vi "waypoint.vi"(11 "Vision Data":dbl[](array[numeric])) -> (3 "Waypoints":dbl[][](array[numeric]))   [LabVIEW 2018]
panel:
  in  "Multiplier":dbl format="%#_13g"
  out "XY Graph":cluster{dbl[], dbl[]}[](graph)
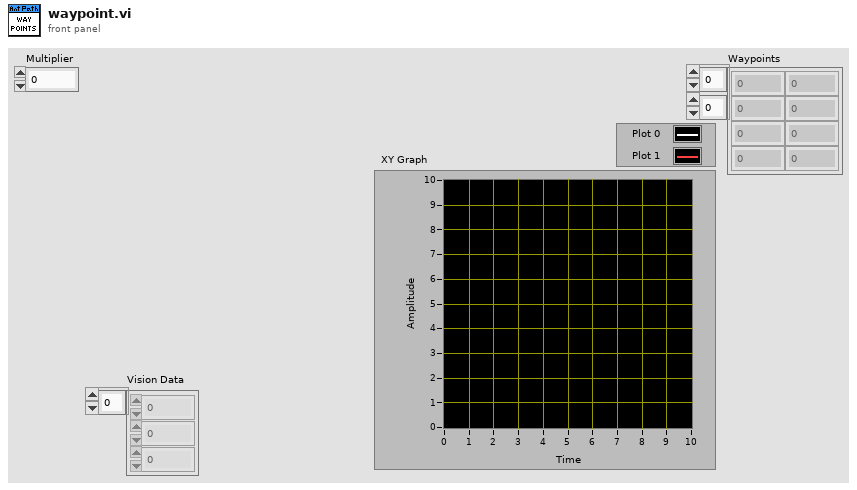
[diagram p1: front panel]
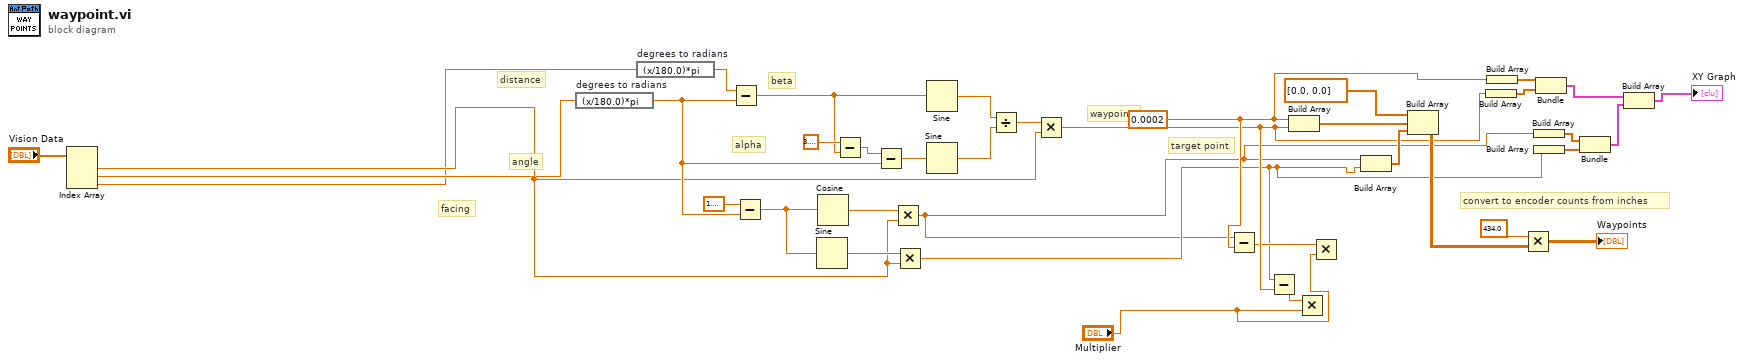
[diagram p0: block diagram]
diagram:
  w7 = 0.0002 ("element")
  # "target point"
  # "waypoint"
  # "facing"
  # "distance"
  # "angle"
  # "convert to encoder counts from inches"
  # "alpha"
  # "beta"
  n1 = Index Array(array="Vision Data") -> (element #1=w10:dbl, element #2=w9:dbl, element #3=w8:dbl)  [unwired: 3 in]
  n2 = expression code="(x/180.0)*pi" "degrees to radians"(w9) -> (w15:dbl)
  n3 = expression code="(x/180.0)*pi" "degrees to radians"(w8) -> (w16:dbl)
  n4 = Subtract(x=w16, y=w15) -> (x-y=w35:dbl)
  n5 = Subtract(x=1.5707963267948966, y=w15) -> (x-y=w27:dbl)
  n6 = Sine(x=w27) -> (sin(x)=w25:dbl)
  n7 = Cosine(x=w27) -> (cos(x)=w26:dbl)
  n8 = Subtract(x=3.141592653589793, y=w35) -> (x-y=w34:dbl)
  n9 = Subtract(x=w34, y=w15) -> (x-y=w33:dbl)
  n10 = Multiply(x=w26, y=w10) -> (x*y=w1:dbl)
  n11 = Multiply(x=w25, y=w10) -> (x*y=w2:dbl)
  n12 = Sine(x=w35) -> (sin(x)=w32:dbl)
  n13 = Sine(x=w33) -> (sin(x)=w31:dbl)
  n14 = Divide(x=w32, y=w31) -> (x/y=w30:dbl)
  n15 = Multiply(x=w30, y=w10) -> (x*y=w6:dbl)
  n16 = Subtract(x=w1, y=w7) -> (x-y=w4:dbl)
  n17 = Subtract(x=w2, y=w6) -> (x-y=w5:dbl)
  n18 = Build Array(w7, w6) -> (w29:dbl[])
  n19 = Multiply(x=w5, y="Multiplier") -> ()  [unwired: 1 out]
  n20 = Multiply(x=w4, y="Multiplier") -> ()  [unwired: 1 out]
  n21 = Build Array(w1, w2) -> (w24:dbl[])
  n22 = Build Array(dbl[] [0.0, 0.0], w29, w24) -> (w14:dbl[][])
  n23 = Build Array(w6) -> (w20:dbl[])
  n24 = Build Array(w7) -> (w21:dbl[])
  n25 = Multiply(x=434.0, y=w14) -> (x*y=→"Waypoints":dbl[][])
  n26 = Build Array(w1) -> (w23:dbl[])
  n27 = Build Array(w2) -> (w22:dbl[])
  n28 = Bundle(w21, w20) -> (w19:cluster{dbl[], dbl[]})  [unwired: 1 in]
  n29 = Bundle(w23, w22) -> (w18:cluster{dbl[], dbl[]})  [unwired: 1 in]
  n30 = Build Array(w19, w18) -> (→"XY Graph":cluster{dbl[], dbl[]}[])
